vi "02 - Interactive.vi"() -> ()   [LabVIEW 2019]
uses:
  Shared/Selection--array.ctl
  Shared/Selection--picture ring.ctl
  Shared/Solution Node--cluster.ctl
  Shared/Solution--picture ring.ctl
  Shared/Direction--enum.ctl
  Shared/Node Type--enum.ctl
  Grassfire/Grassfire.lvclass
  Shared/Shared.lvlib
panel:
  in  "Preset Grid 5":bool
  in  "Optimised":bool=TRUE
  in  "Preset Grid 4":bool
  out "Error Out":errorcluster
  in  "Get Directions":bool=TRUE
  in  "Preset Grid 3":bool
  in  "Preset Grid 2":bool
  in  "Calculate":bool
  in  "Preset Grid 1":bool
  in  "Tab":enum32{"Selection", "Solution"}(tab)
  in  "Selection Grid":T1
  in  "Heading":T3
  out "Solution Grid":T4[][](array[typedef])
  out "Directions":T3[](array[typedef])
  out "ms":u32
  # "1. Run VI\n2. Edit the Selection Grid and select Heading\n     Heading is the direction the Robot is facing\n3. Click \"Calculate\"\n    Enabled when only 1 start and 1 end node exist.\n4. Observe Solution Grid"
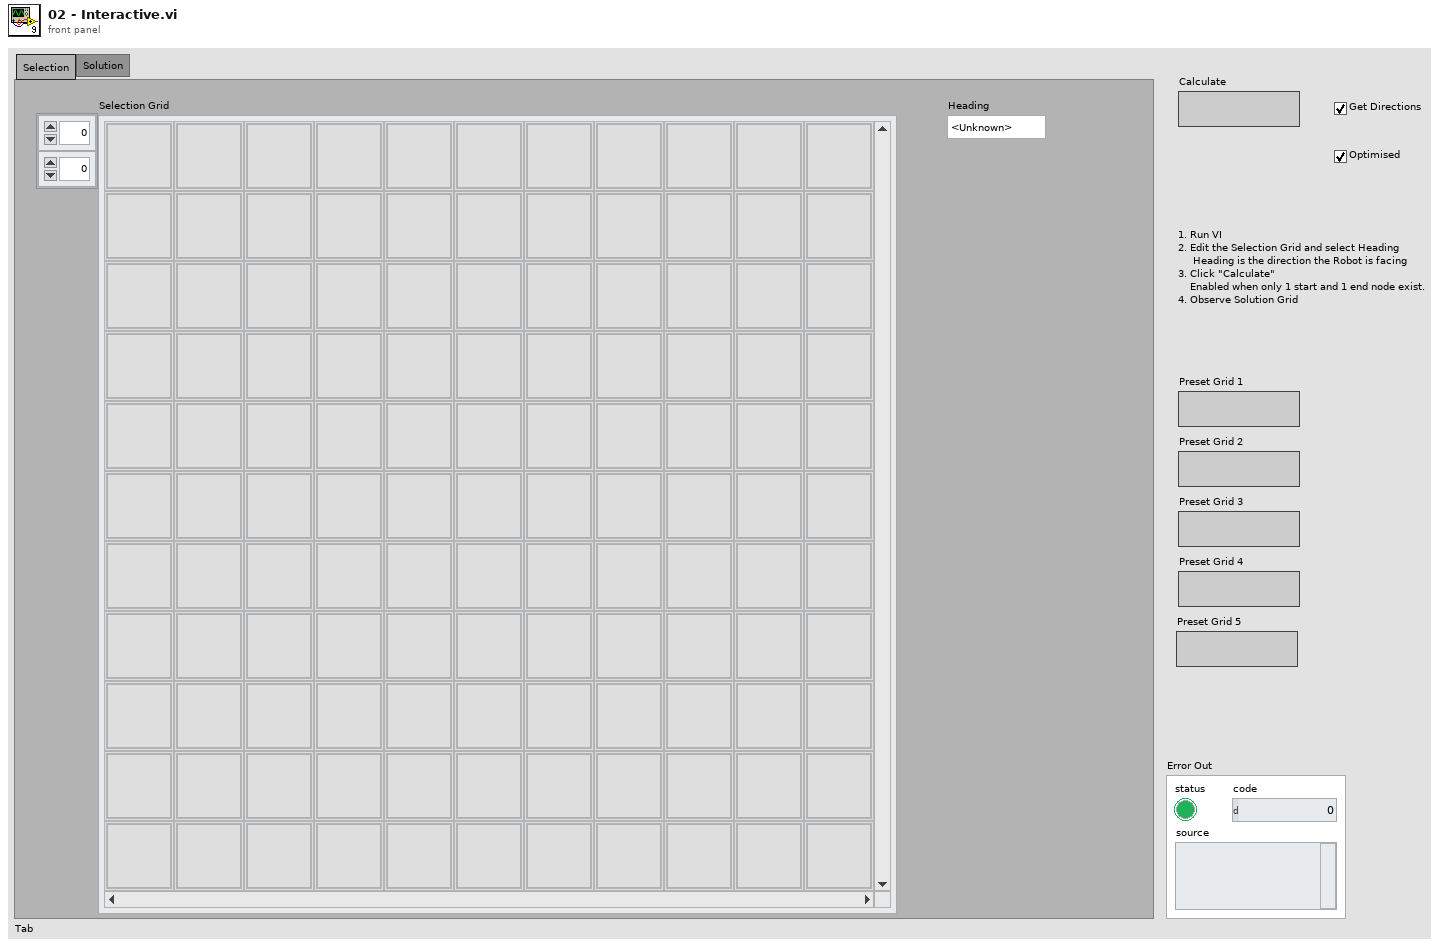
[diagram p1: front panel]
types:
  T1 = typedef "Shared.lvlib/Selection--array.ctl" = cluster{"Grid Value":T2}[][]
  T2 = typedef "Shared.lvlib/Selection--picture ring.ctl" = i64
  T3 = typedef "Shared.lvlib/Direction--enum.ctl" = enum16{"<Unknown>", "Right", "Down", "Left", "Up"}
  T4 = typedef "Shared.lvlib/Solution Node--cluster.ctl" = cluster{"Type":T5, "Distance":string}
  T5 = typedef "Shared.lvlib/Solution--picture ring.ctl" = i64
  T6 = enum8{"Enabled", "Disabled", "Disabled and Grayed Out"}
  T7 = typedef "Shared.lvlib/Node Type--enum.ctl" = enum16{"Empty", "Blocked", "Start", "End", "Path"}
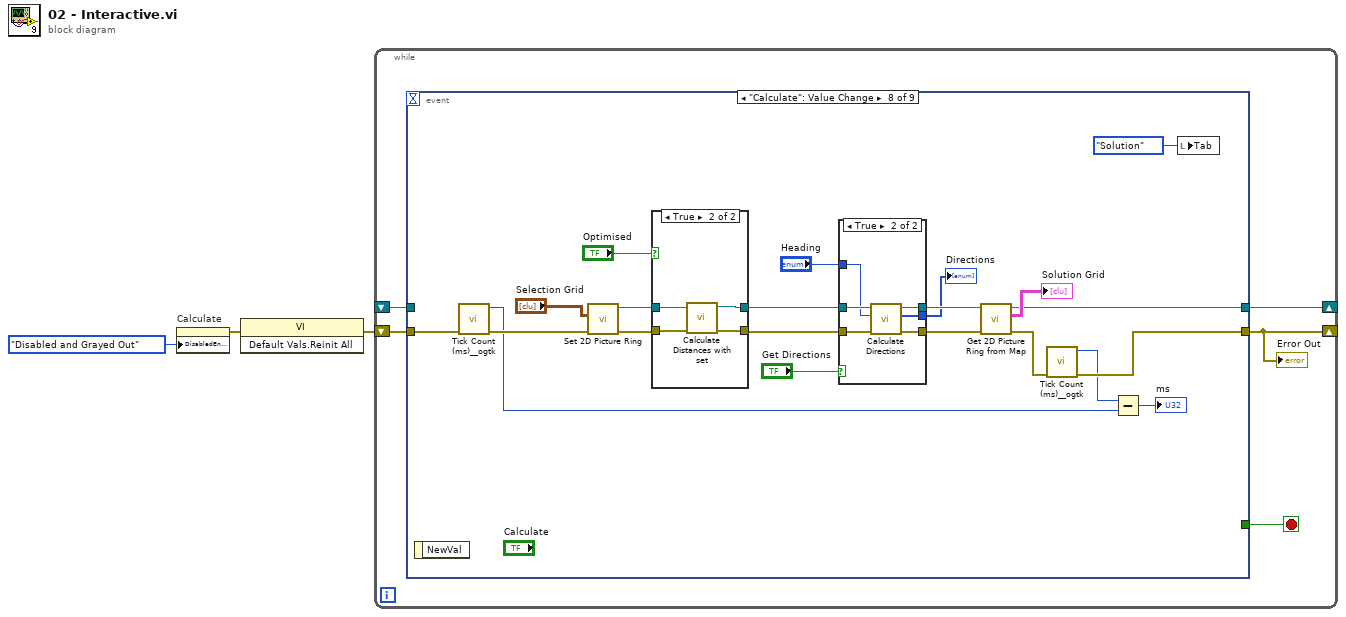
[diagram p0: block diagram]
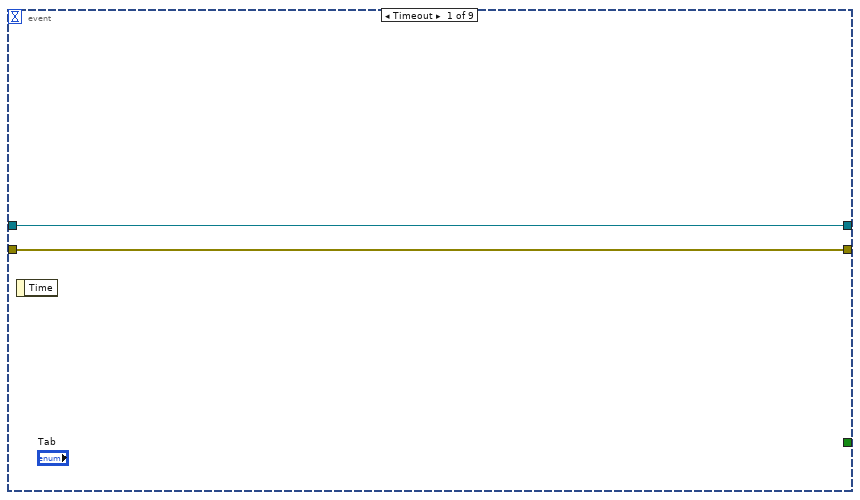
[diagram p2: hidden frame]
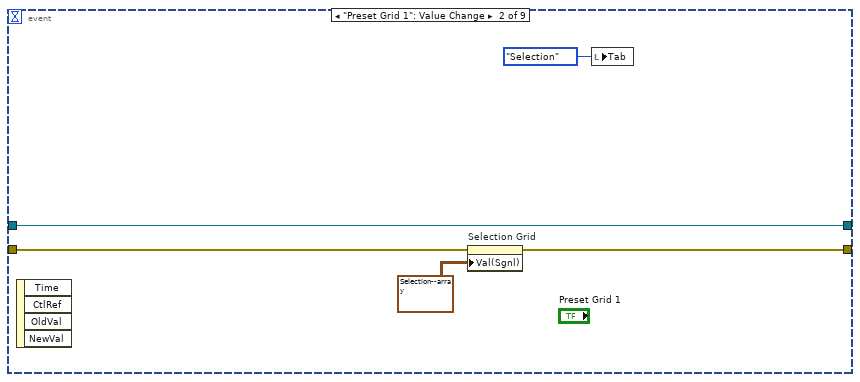
[diagram p3: hidden frame]
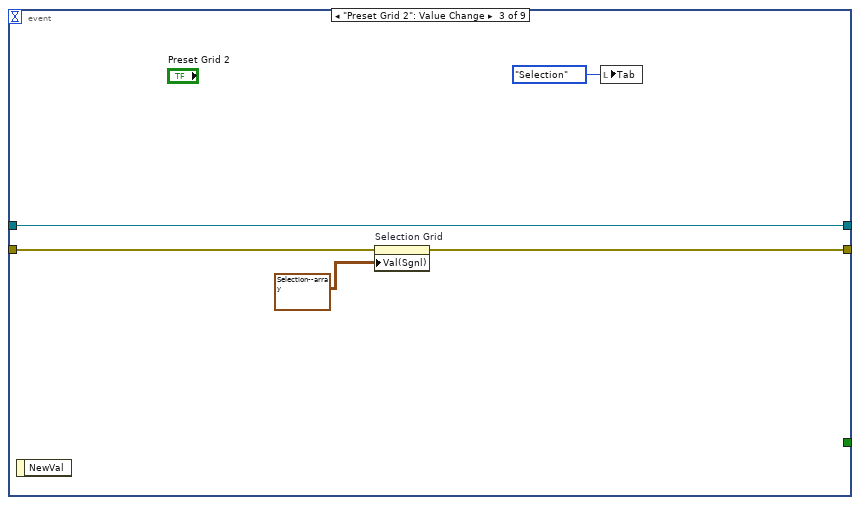
[diagram p4: hidden frame]
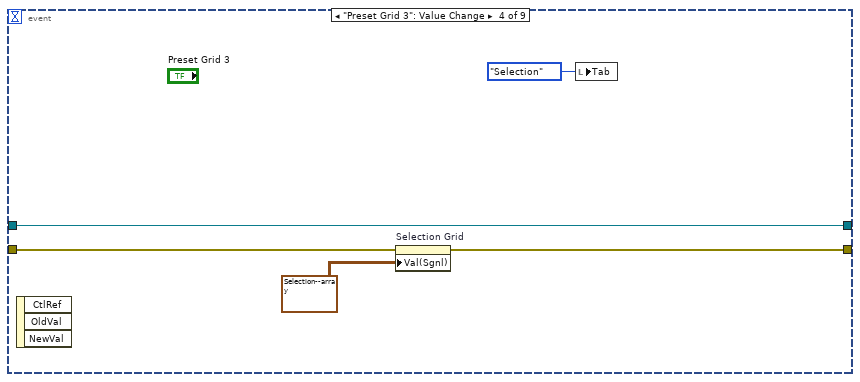
[diagram p5: hidden frame]
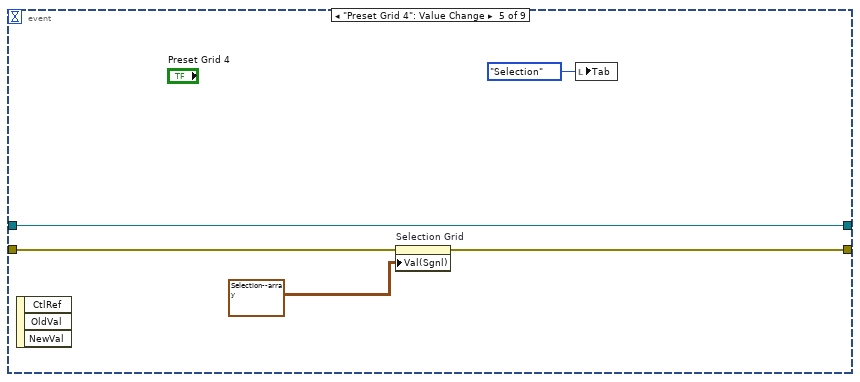
[diagram p6: hidden frame]
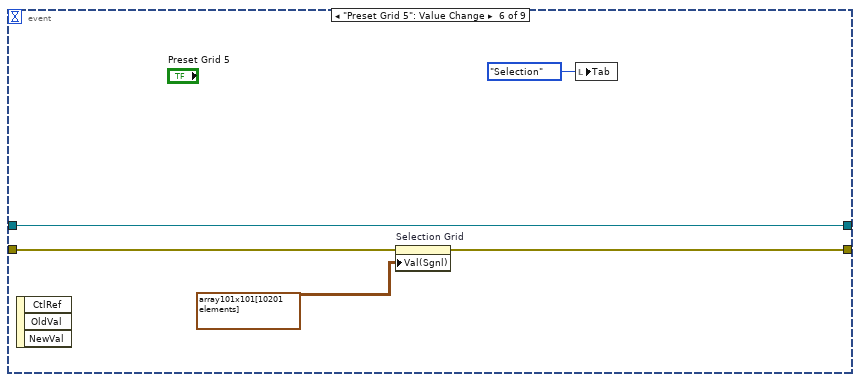
[diagram p7: hidden frame]
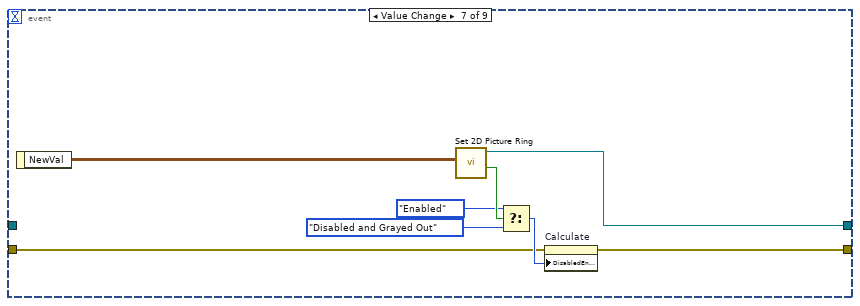
[diagram p8: hidden frame]
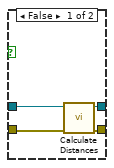
[diagram p9: hidden frame]
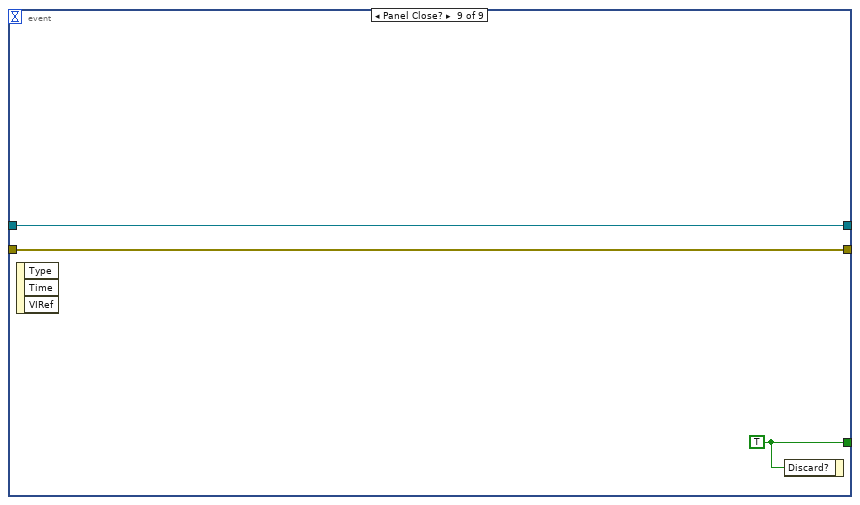
[diagram p11: hidden frame]
diagram:
  n1 = property on="Calculate" class="Bool"("DisabledEnum"=T6."Disabled and Grayed Out" ("f")) -> (error out=w2:errorcluster)  [unwired: 2 in, 1 out]
  n2 = invoke class="VI" method="Default Vals.Reinit All"(error in=w2) -> (error out=w1:errorcluster)  [unwired: 2 in, 2 out]
  n3 = while {
    shift-right: [w7] -> _
    shift-left: _ -> [w6]
    shift-right: [w4] -> _
    shift-left: w1 -> [w5]
    stop <- w8 stop-if-true
    n4 = event shown="[7] \"Calculate\": Value Change" {
      selector: _ -> [_ _ _ _ _ _ _ _ _]
      dyn-events: _ -> [_ _ _ _ _ _ _ _ _]
      timeout: _ -> [_ _ _ _ _ _ _ _ _]
      tunnel: [_ _ _ _ _ _ _ _ w83] -> w8
      tunnel: [w10 w15 w20 w25 w30 w35 w38 w60 w82] -> w7
      tunnel: w6 -> [w10 w15 w20 w25 w30 w35 _ _ w82]
      tunnel: [w9 w11 w16 w21 w27 w32 w36 w48 w81] -> w4
      tunnel: w5 -> [w9 w12 w17 w22 w28 w33 w37 w51 w81]
      event Timeout {
        n5 = event-data() -> ()  [unwired: 1 in, 1 out]
      }
      event "Preset Grid 1": Value Change {
        n6 = event-data() -> ()  [unwired: 1 in, 4 out]
        n7 = property on="Selection Grid" class="Arr (strict)"(error in=w12, "Val(Sgnl)"=T1 [[{"Grid Value"=0}, {"Grid Value"=2}, {"Grid Value"=0}, {"Grid Value"=0}, {"Grid Value"=0}], [{"Grid Value"=0}, {"Grid Value"=1}, {"Grid Value"=0}, {"Grid Value"=0}, {"Grid Value"=0}], [{"Grid Value"=0}, {"Grid Value"=0}, {"Grid Value"=1}, {"Grid Value"=0}, {"Grid Value"=0}], [{"Grid Value"=0}, {"Grid Value"=0}, {"Grid Value"=0}, {"Grid Value"=3}, {"Grid Value"=0}], [{"Grid Value"=0}, {"Grid Value"=0}, {"Grid Value"=0}, {"Grid Value"=0}, {"Grid Value"=0}]] ("Value (Signaling)")) -> (error out=w11:errorcluster)  [unwired: 1 in, 1 out]
        n8 = local write "Tab"(enum32{"Selection", "Solution"}."Selection" ("Tab")) -> ()
      }
      event "Preset Grid 2": Value Change {
        n9 = event-data() -> ()  [unwired: 1 in, 1 out]
        n10 = property on="Selection Grid" class="Arr (strict)"(error in=w17, "Val(Sgnl)"=T1 [[{"Grid Value"=0}, {"Grid Value"=0}, {"Grid Value"=0}, {"Grid Value"=0}, {"Grid Value"=0}, {"Grid Value"=0}, {"Grid Value"=0}, {"Grid Value"=0}, {"Grid Value"=0}, {"Grid Value"=0}, {"Grid Value"=0}], [{"Grid Value"=0}, {"Grid Value"=0}, {"Grid Value"=0}, {"Grid Value"=0}, {"Grid Value"=0}, {"Grid Value"=0}, {"Grid Value"=0}, {"Grid Value"=0}, {"Grid Value"=0}, {"Grid Value"=0}, {"Grid Value"=0}], [{"Grid Value"=0}, {"Grid Value"=0}, {"Grid Value"=2}, {"Grid Value"=0}, {"Grid Value"=0}, {"Grid Value"=0}, {"Grid Value"=0}, {"Grid Value"=0}, {"Grid Value"=0}, {"Grid Value"=0}, {"Grid Value"=0}], [{"Grid Value"=0}, {"Grid Value"=0}, {"Grid Value"=0}, {"Grid Value"=0}, {"Grid Value"=0}, {"Grid Value"=0}, {"Grid Value"=0}, {"Grid Value"=0}, {"Grid Value"=0}, {"Grid Value"=0}, {"Grid Value"=0}], [{"Grid Value"=0}, {"Grid Value"=0}, {"Grid Value"=0}, {"Grid Value"=0}, {"Grid Value"=0}, {"Grid Value"=0}, {"Grid Value"=0}, {"Grid Value"=0}, {"Grid Value"=0}, {"Grid Value"=0}, {"Grid Value"=0}], [{"Grid Value"=0}, {"Grid Value"=0}, {"Grid Value"=0}, {"Grid Value"=0}, {"Grid Value"=0}, {"Grid Value"=0}, {"Grid Value"=0}, {"Grid Value"=0}, {"Grid Value"=0}, {"Grid Value"=0}, {"Grid Value"=0}], [{"Grid Value"=0}, {"Grid Value"=0}, {"Grid Value"=0}, {"Grid Value"=0}, {"Grid Value"=0}, {"Grid Value"=0}, {"Grid Value"=0}, {"Grid Value"=0}, {"Grid Value"=0}, {"Grid Value"=0}, {"Grid Value"=0}], [{"Grid Value"=0}, {"Grid Value"=0}, {"Grid Value"=0}, {"Grid Value"=0}, {"Grid Value"=1}, {"Grid Value"=1}, {"Grid Value"=1}, {"Grid Value"=1}, {"Grid Value"=1}, {"Grid Value"=1}, {"Grid Value"=1}], [{"Grid Value"=0}, {"Grid Value"=0}, {"Grid Value"=0}, {"Grid Value"=0}, {"Grid Value"=1}, {"Grid Value"=0}, {"Grid Value"=0}, {"Grid Value"=0}, {"Grid Value"=0}, {"Grid Value"=0}, {"Grid Value"=0}], [{"Grid Value"=0}, {"Grid Value"=0}, {"Grid Value"=0}, {"Grid Value"=0}, {"Grid Value"=1}, {"Grid Value"=0}, {"Grid Value"=0}, {"Grid Value"=3}, {"Grid Value"=0}, {"Grid Value"=0}, {"Grid Value"=0}], [{"Grid Value"=0}, {"Grid Value"=0}, {"Grid Value"=0}, {"Grid Value"=0}, {"Grid Value"=1}, {"Grid Value"=0}, {"Grid Value"=0}, {"Grid Value"=0}, {"Grid Value"=0}, {"Grid Value"=0}, {"Grid Value"=0}]] ("Selection Grid")) -> (error out=w16:errorcluster)  [unwired: 1 in, 1 out]
        n11 = local write "Tab"(enum32{"Selection", "Solution"}."Selection" ("Tab")) -> ()
      }
      event "Preset Grid 3": Value Change {
        n12 = event-data() -> ()  [unwired: 1 in, 3 out]
        n13 = property on="Selection Grid" class="Arr (strict)"(error in=w22, "Val(Sgnl)"=T1 [[{"Grid Value"=0}, {"Grid Value"=0}, {"Grid Value"=0}, {"Grid Value"=0}, {"Grid Value"=0}, {"Grid Value"=0}, {"Grid Value"=0}, {"Grid Value"=0}, {"Grid Value"=0}, {"Grid Value"=0}, {"Grid Value"=0}], [{"Grid Value"=0}, {"Grid Value"=0}, {"Grid Value"=0}, {"Grid Value"=0}, {"Grid Value"=0}, {"Grid Value"=0}, {"Grid Value"=0}, {"Grid Value"=0}, {"Grid Value"=1}, {"Grid Value"=1}, {"Grid Value"=0}], [{"Grid Value"=0}, {"Grid Value"=0}, {"Grid Value"=2}, {"Grid Value"=0}, {"Grid Value"=0}, {"Grid Value"=0}, {"Grid Value"=0}, {"Grid Value"=0}, {"Grid Value"=1}, {"Grid Value"=0}, {"Grid Value"=0}], [{"Grid Value"=0}, {"Grid Value"=0}, {"Grid Value"=0}, {"Grid Value"=0}, {"Grid Value"=0}, {"Grid Value"=0}, {"Grid Value"=0}, {"Grid Value"=0}, {"Grid Value"=0}, {"Grid Value"=0}, {"Grid Value"=0}], [{"Grid Value"=0}, {"Grid Value"=0}, {"Grid Value"=0}, {"Grid Value"=0}, {"Grid Value"=0}, {"Grid Value"=0}, {"Grid Value"=0}, {"Grid Value"=0}, {"Grid Value"=0}, {"Grid Value"=0}, {"Grid Value"=0}], [{"Grid Value"=0}, {"Grid Value"=0}, {"Grid Value"=0}, {"Grid Value"=0}, {"Grid Value"=0}, {"Grid Value"=1}, {"Grid Value"=0}, {"Grid Value"=1}, {"Grid Value"=0}, {"Grid Value"=0}, {"Grid Value"=0}], [{"Grid Value"=0}, {"Grid Value"=0}, {"Grid Value"=0}, {"Grid Value"=0}, {"Grid Value"=1}, {"Grid Value"=1}, {"Grid Value"=0}, {"Grid Value"=1}, {"Grid Value"=0}, {"Grid Value"=0}, {"Grid Value"=0}], [{"Grid Value"=0}, {"Grid Value"=1}, {"Grid Value"=1}, {"Grid Value"=0}, {"Grid Value"=1}, {"Grid Value"=1}, {"Grid Value"=0}, {"Grid Value"=1}, {"Grid Value"=1}, {"Grid Value"=1}, {"Grid Value"=0}], [{"Grid Value"=0}, {"Grid Value"=0}, {"Grid Value"=0}, {"Grid Value"=0}, {"Grid Value"=0}, {"Grid Value"=0}, {"Grid Value"=0}, {"Grid Value"=0}, {"Grid Value"=0}, {"Grid Value"=0}, {"Grid Value"=0}], [{"Grid Value"=0}, {"Grid Value"=0}, {"Grid Value"=0}, {"Grid Value"=0}, {"Grid Value"=0}, {"Grid Value"=0}, {"Grid Value"=0}, {"Grid Value"=3}, {"Grid Value"=0}, {"Grid Value"=0}, {"Grid Value"=0}], [{"Grid Value"=0}, {"Grid Value"=0}, {"Grid Value"=0}, {"Grid Value"=0}, {"Grid Value"=0}, {"Grid Value"=0}, {"Grid Value"=0}, {"Grid Value"=0}, {"Grid Value"=0}, {"Grid Value"=0}, {"Grid Value"=0}]] ("Selection Grid")) -> (error out=w21:errorcluster)  [unwired: 1 in, 1 out]
        n14 = local write "Tab"(enum32{"Selection", "Solution"}."Selection" ("Tab")) -> ()
      }
      event "Preset Grid 4": Value Change {
        n15 = event-data() -> ()  [unwired: 1 in, 3 out]
        n16 = property on="Selection Grid" class="Arr (strict)"(error in=w28, "Val(Sgnl)"=T1 [[{"Grid Value"=0}, {"Grid Value"=2}, {"Grid Value"=0}, {"Grid Value"=1}, {"Grid Value"=0}, {"Grid Value"=0}, {"Grid Value"=0}, {"Grid Value"=0}, {"Grid Value"=0}, {"Grid Value"=1}, {"Grid Value"=0}], [{"Grid Value"=0}, {"Grid Value"=1}, {"Grid Value"=0}, {"Grid Value"=0}, {"Grid Value"=0}, {"Grid Value"=1}, {"Grid Value"=1}, {"Grid Value"=1}, {"Grid Value"=0}, {"Grid Value"=0}, {"Grid Value"=0}], [{"Grid Value"=0}, {"Grid Value"=0}, {"Grid Value"=1}, {"Grid Value"=0}, {"Grid Value"=1}, {"Grid Value"=0}, {"Grid Value"=1}, {"Grid Value"=0}, {"Grid Value"=0}, {"Grid Value"=1}, {"Grid Value"=0}], [{"Grid Value"=1}, {"Grid Value"=0}, {"Grid Value"=0}, {"Grid Value"=0}, {"Grid Value"=1}, {"Grid Value"=1}, {"Grid Value"=1}, {"Grid Value"=0}, {"Grid Value"=1}, {"Grid Value"=0}, {"Grid Value"=0}], [{"Grid Value"=0}, {"Grid Value"=0}, {"Grid Value"=1}, {"Grid Value"=1}, {"Grid Value"=0}, {"Grid Value"=0}, {"Grid Value"=0}, {"Grid Value"=0}, {"Grid Value"=1}, {"Grid Value"=0}, {"Grid Value"=1}], [{"Grid Value"=0}, {"Grid Value"=1}, {"Grid Value"=1}, {"Grid Value"=0}, {"Grid Value"=0}, {"Grid Value"=0}, {"Grid Value"=1}, {"Grid Value"=1}, {"Grid Value"=0}, {"Grid Value"=1}, {"Grid Value"=0}], [{"Grid Value"=0}, {"Grid Value"=0}, {"Grid Value"=1}, {"Grid Value"=0}, {"Grid Value"=1}, {"Grid Value"=1}, {"Grid Value"=1}, {"Grid Value"=0}, {"Grid Value"=0}, {"Grid Value"=0}, {"Grid Value"=0}], [{"Grid Value"=1}, {"Grid Value"=0}, {"Grid Value"=1}, {"Grid Value"=0}, {"Grid Value"=0}, {"Grid Value"=0}, {"Grid Value"=1}, {"Grid Value"=0}, {"Grid Value"=1}, {"Grid Value"=1}, {"Grid Value"=1}], [{"Grid Value"=0}, {"Grid Value"=0}, {"Grid Value"=1}, {"Grid Value"=0}, {"Grid Value"=1}, {"Grid Value"=0}, {"Grid Value"=1}, {"Grid Value"=0}, {"Grid Value"=0}, {"Grid Value"=0}, {"Grid Value"=1}], [{"Grid Value"=0}, {"Grid Value"=1}, {"Grid Value"=1}, {"Grid Value"=0}, {"Grid Value"=1}, {"Grid Value"=0}, {"Grid Value"=0}, {"Grid Value"=0}, {"Grid Value"=1}, {"Grid Value"=3}, {"Grid Value"=0}], [{"Grid Value"=0}, {"Grid Value"=0}, {"Grid Value"=0}, {"Grid Value"=0}, {"Grid Value"=1}, {"Grid Value"=0}, {"Grid Value"=0}, {"Grid Value"=0}, {"Grid Value"=1}, {"Grid Value"=0}, {"Grid Value"=0}]] ("Selection Grid")) -> (error out=w27:errorcluster)  [unwired: 1 in, 1 out]
        n17 = local write "Tab"(enum32{"Selection", "Solution"}."Selection" ("Tab")) -> ()
      }
      event "Preset Grid 5": Value Change {
        n18 = event-data() -> ()  [unwired: 1 in, 3 out]
        n19 = property on="Selection Grid" class="Arr (strict)"(error in=w33, "Val(Sgnl)"=cluster{"Type":T7}[][] array101x101[10201 elements]) -> (error out=w32:errorcluster)  [unwired: 1 in, 1 out]
        n20 = local write "Tab"(enum32{"Selection", "Solution"}."Selection" ("Tab")) -> ()
      }
      event Value Change {
        n21 = event-data() -> ("NewVal"=w43:T1)  [unwired: 1 in]
        n22 = call "Set 2D Picture Ring.vi"("Selection Grid"=w43) -> ("Valid"=w42:bool, "Grassfire out"=w38:refnum<class "Grassfire.lvclass">)  [unwired: 8 in, 1 out]
        n23 = Select(t=T6."Enabled" ("Disabled"), s=w42, f=T6."Disabled and Grayed Out") -> (s? t:f=w40:T6)
        n24 = property on="Calculate" class="Bool"(error in=w37, "DisabledEnum"=w40) -> (error out=w36:errorcluster)  [unwired: 1 in, 1 out]
      }
      event "Calculate": Value Change {
        n25 = event-data() -> ()  [unwired: 1 in, 1 out]
        n26 = call <userlib>:"Tick Count (ms)__ogtk.vi"("error in (no error)"=w51) -> ("error out"=w50:errorcluster, "millisecond timer value"=w46:u32)  [unwired: 9 in]
        n27 = call "Set 2D Picture Ring.vi"("error in (no error)"=w50, "Selection Grid"="Selection Grid") -> ("error out"=w54:errorcluster, "Grassfire out"=w55:refnum<class "Grassfire.lvclass">)  [unwired: 7 in, 1 out]
        n28 = case shown="True" "Optimised" {
          tunnel: [w68 w71] -> w64
          tunnel: [w67 w69] -> w58
          tunnel: w55 -> [w66 w72]
          tunnel: w54 -> [w65 w70]
          frame False {
            n29 = call-dynamic "Calculate Distances.vi"("error in (no error)"=w65, "Grassfire in"=w66) -> ("error out"=w67:errorcluster, "Grassfire out"=w68:refnum<class "Grassfire.lvclass">)  [unwired: 8 in]
          }
          frame True {
            n30 = call-dynamic "Calculate Distances with set.vi"("error in (no error)"=w70, "Grassfire in"=w72) -> ("error out"=w69:errorcluster, "Grassfire out"=w71:refnum<class "Grassfire.lvclass">)  [unwired: 8 in]
          }
        }
        n31 = case shown="True" "Get Directions" {
          tunnel: w64 -> [w74 w80]
          tunnel: [w74 w79] -> w63
          tunnel: [_ w78] -> w52
          tunnel: "Heading" -> [_ w77]
          tunnel: w58 -> [w73 w76]
          tunnel: [w73 w75] -> w57
          frame False {
          }
          frame True {
            n32 = call-dynamic "Calculate Directions.vi"("error in (no error)"=w76, "Heading"=w77, "Grassfire in"=w80) -> ("error out"=w75:errorcluster, "Directions"=w78:T3[], "Grassfire out"=w79:refnum<class "Grassfire.lvclass">)  [unwired: 6 in]
          }
        }
        "Directions" <- w52
        n33 = call-dynamic "Get 2D Picture Ring from Map.vi"("error in (no error)"=w57, "Grassfire in"=w63) -> ("error out"=w49:errorcluster, "Array"=→"Solution Grid":T4[][], "Grassfire out"=w60:refnum<class "Grassfire.lvclass">)  [unwired: 7 in]
        n34 = call <userlib>:"Tick Count (ms)__ogtk.vi"("error in (no error)"=w49) -> ("error out"=w48:errorcluster, "millisecond timer value"=w47:u32)  [unwired: 9 in]
        n35 = Subtract(x=w47, y=w46) -> (x-y=→"ms":u32)
        n36 = local write "Tab"(enum32{"Selection", "Solution"}."Solution" ("Tab")) -> ()
      }
      event Panel Close? {
        w83 = TRUE ("Discard?")
        n37 = event-data() -> ()  [unwired: 1 in, 3 out]
        n38 = event-data("Discard?"=w83) -> ()  [unwired: 1 in, 1 out]
      }
    }
    "Error Out" <- w4
  }
